vi "subGetNodeQualifiedNames.vi"(8 "error in (no error)":errorcluster, 9 "Parent node":string, 11 "node[] in":refnum<k20>[](array[refnum])) -> (0 "error out":errorcluster, 1 "node name[]":string[](array[string]), 3 "node[]":refnum<k20>[](array[refnum]))   [LabVIEW 2020, in "DefaultExtensions.lvlib" / "CDefaultRuleFileParser.lvclass"]
uses:
  CDefaultRuleFileParser.lvclass
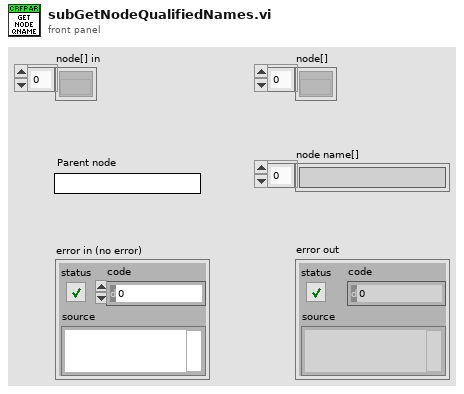
[diagram p1: front panel]
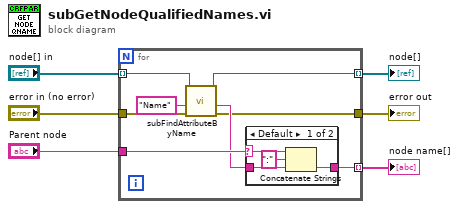
[diagram p0: block diagram]
diagram:
  n1 = for {
    tunnel: "error in (no error)" -> [w14]
    tunnel: "node[] in" -> [w12] mode=indexing
    tunnel: "Parent node" -> [w11]
    tunnel: [w9] -> w2 mode=indexing
    tunnel: [w8] -> w6 mode=indexing
    tunnel: [w7] -> w4
    n2 = call "subFindAttributeByName.vi"("error in (no error)"=w14, "key"="Name", "Node Reg in"=w12) -> ("error out"=w7:errorcluster, "value"=w10:string, "Node Reg"=w9:refnum<k20>)  [unwired: 5 in, 1 out]
    n3 = case shown="Default" w11 {
      selector: w11 -> [w18 _]
      tunnel: w10 -> [w17 w19]
      tunnel: [w15 w19] -> w8
      frame Default {
        n4 = Concatenate Strings(w18, ":" ("string"), w17) -> (w15:string)
      }
      frame "" {
      }
    }
  }
  "node name[]" <- w6
  "node[]" <- w2
  "error out" <- w4
